vi "De-Initialize.vi"(8 "error in (no error)":errorcluster, 11 "Ni-Scope Digitizer in":refnum<class "Ni-Scope Digitizer.lvclass">) -> (0 "error out":errorcluster, 3 "Ni-Scope Digitizer out":refnum<class "Ni-Scope Digitizer.lvclass">)   [LabVIEW 2016, in "Ni-Scope Digitizer.lvclass"]
uses:
  Ni-Scope Digitizer.lvclass
  Ni-Scope Digitizer.lvclass/Ni-Scope Digitizer.ctl
  Instruments/Pulse Driver/Pulse Driver.lvclass
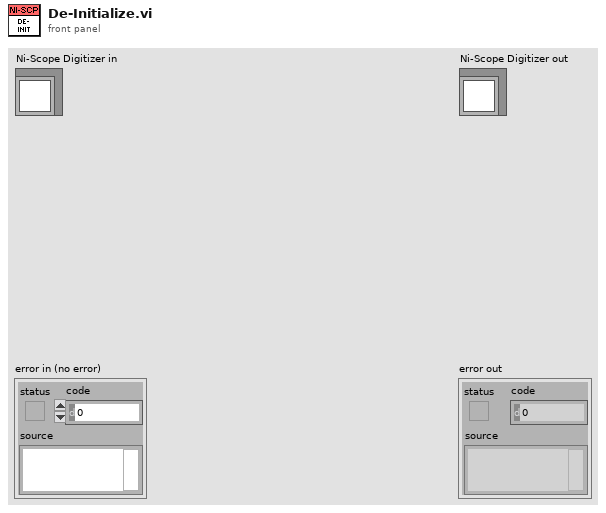
[diagram p1: front panel]
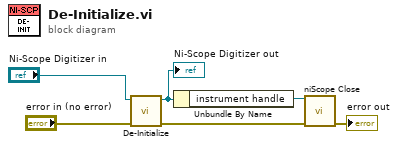
[diagram p0: block diagram]
diagram:
  n1 = call-parent "De-Initialize.vi"("error in (no error)"="error in (no error)", "Instrument Driver in"="Ni-Scope Digitizer in") -> ("error out"=w3:errorcluster, "Instrument Driver out"=w1:refnum<class "Ni-Scope Digitizer.lvclass">)  [unwired: 8 in]
  "Ni-Scope Digitizer out" <- w1
  n2 = Unbundle By Name(w1) -> ("instrument handle"=w6:refnum<k15>)
  n3 = call <instrlib>:"niScope Close.vi"("instrument handle"=w6, "error in"=w3) -> ("error out"=→"error out":errorcluster)  [unwired: 13 in]
